vi "TimeStampToDateTimeInt.vi"(0 "Time Stamp":timestamp=timestamp(3357882633.0878906 s since 1904-01-01)) -> (1 "timeInt":u32, 2 "dateInt":u16)   [LabVIEW 2009]
panel:
  out "number":u32
  out "milliseconds":string
  out "seconds":string
  out "minute":string
  out "hour":string
  out "year":string
  out "month":string
  out "day":string
  out "time":string
  out "date":string
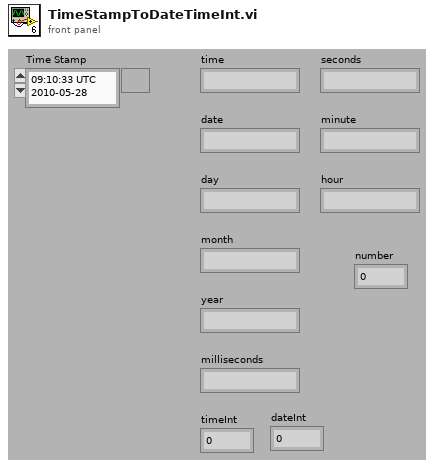
[diagram p1: front panel]
types:
  T1 = cluster{"Boolean array[0]":bool, "Boolean array[1]":bool, "Boolean array[2]":bool, "Boolean array[3]":bool, "Boolean array[4]":bool, "Boolean array[5]":bool, "Boolean array[6]":bool, "Boolean array[7]":bool, "Boolean array[8]":bool, "Boolean array[9]":bool}
  T2 = cluster{"Boolean array[0]":bool, "Boolean array[1]":bool, "Boolean array[2]":bool, "Boolean array[3]":bool, "Boolean array[4]":bool, "Boolean array[5]":bool}
  T3 = cluster{"Boolean array[0]":bool, "Boolean array[1]":bool, "Boolean array[2]":bool, "Boolean array[3]":bool, "Boolean array[4]":bool}
  T4 = cluster{"Boolean array[0]":bool, "Boolean array[1]":bool, "Boolean array[2]":bool, "Boolean array[3]":bool}
  T5 = cluster{"Boolean array[0]":bool, "Boolean array[1]":bool, "Boolean array[2]":bool, "Boolean array[3]":bool, "Boolean array[4]":bool, "Boolean array[5]":bool, "Boolean array[6]":bool}
  T6 = cluster{"Boolean array[0]":bool, "Boolean array[1]":bool, "Boolean array[2]":bool, "Boolean array[3]":bool, "Boolean array[4]":bool, "Boolean array[5]":bool, "Boolean array[6]":bool, "Boolean array[7]":bool, "Boolean array[8]":bool, "Boolean array[9]":bool, "Boolean array[0]":bool, "Boolean array[1]":bool, "Boolean array[2]":bool, "Boolean array[3]":bool, "Boolean array[4]":bool, "Boolean array[5]":bool, "Boolean array[0]":bool, "Boolean array[1]":bool, "Boolean array[2]":bool, "Boolean array[3]":bool, "Boolean array[4]":bool, "Boolean array[5]":bool, "Boolean array[0]":bool, "Boolean array[1]":bool, "Boolean array[2]":bool, "Boolean array[3]":bool, "Boolean array[4]":bool, "Boolean array[0]":bool, "Boolean array[1]":bool, "Boolean array[2]":bool, "Boolean array[3]":bool, "Boolean array[4]":bool}
  T7 = cluster{"Boolean array[0]":bool, "Boolean array[1]":bool, "Boolean array[2]":bool, "Boolean array[3]":bool, "Boolean array[4]":bool, "Boolean array[0]":bool, "Boolean array[1]":bool, "Boolean array[2]":bool, "Boolean array[3]":bool, "Boolean array[0]":bool, "Boolean array[1]":bool, "Boolean array[2]":bool, "Boolean array[3]":bool, "Boolean array[4]":bool, "Boolean array[5]":bool, "Boolean array[6]":bool}
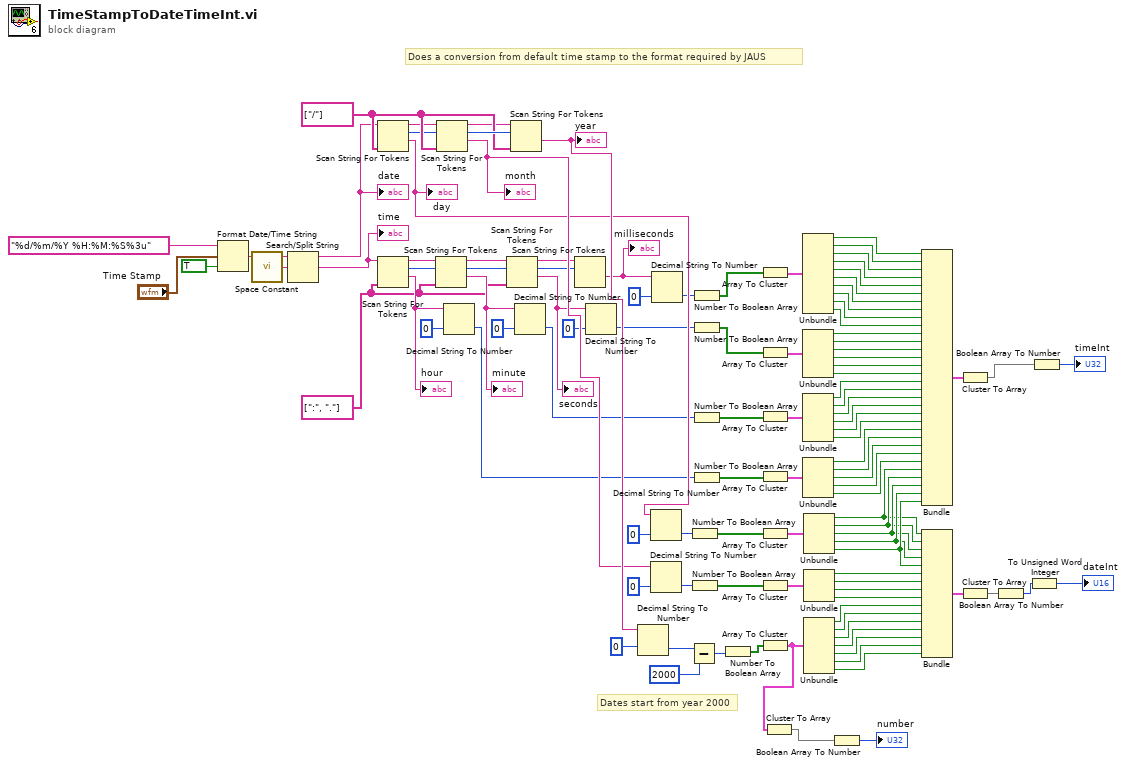
[diagram p0: block diagram]
diagram:
  w25 = string[] [":", "."] ("delimiters (\\s,\\t,\\r,\\n)")
  w18 = string[] ["/"] ("delimiters (\\s,\\t,\\r,\\n)")
  # "Dates start from year 2000"
  # "Does a conversion from default time stamp to the format required by JAUS"
  n1 = Format Date/Time String(time format string (%c)="%d/%m/%Y %H:%M:%S%3u", seconds (now)="Time Stamp", UTC format=TRUE) -> (date/time string=w12:string)
  n2 = call <vilib>:"Space Constant.vi"() -> ("String"=w13:string)
  n3 = Search/Split String(string=w12, search string/char (-)=w13) -> (substring before match=w14:string, match + rest of string=w24:string)  [unwired: 1 in, 1 out]
  "date" <- w14
  "time" <- w24
  n4 = Scan String For Tokens(6:w18, 9:w14) -> (1:w76:string, 2:w16:i32, 3:w15:string)  [unwired: 4 in, 1 out]
  "day" <- w76
  n5 = Scan String For Tokens(6:w25, 9:w24) -> (1:w28:string, 2:w21:i32, 3:w20:string)  [unwired: 4 in, 1 out]
  "hour" <- w28
  n6 = Scan String For Tokens(6:w25, 8:w21, 9:w20) -> (1:w34:string, 2:w23:i32, 3:w22:string)  [unwired: 3 in, 1 out]
  "minute" <- w34
  n7 = Scan String For Tokens(6:w18, 8:w16, 9:w15) -> (1:w91:string, 2:w19:i32, 3:w17:string)  [unwired: 3 in, 1 out]
  "month" <- w91
  n8 = Decimal String To Number(string=w28, default (0L)=u8 0 ("default (0 I32)")) -> (number=w30:u8)  [unwired: 1 in, 1 out]
  n9 = Scan String For Tokens(6:w25, 8:w23, 9:w22) -> (1:w39:string, 2:w27:i32, 3:w26:string)  [unwired: 3 in, 1 out]
  "seconds" <- w39
  n10 = Scan String For Tokens(6:w18, 8:w19, 9:w17) -> (1:w97:string)  [unwired: 3 in, 3 out]
  "year" <- w97
  n11 = Decimal String To Number(string=w34, default (0L)=u8 0 ("default (0 I32)")) -> (number=w32:u8)  [unwired: 1 in, 1 out]
  n12 = Scan String For Tokens(8:w27, 9:w26) -> (1:w43:string)  [unwired: 4 in, 3 out]
  "milliseconds" <- w43
  n13 = Decimal String To Number(string=w39, default (0L)=u8 0 ("default (0 I32)")) -> (number=w36:u8)  [unwired: 1 in, 1 out]
  n14 = Decimal String To Number(string=w97, default (0L)=u16 0 ("default (0 I32)")) -> (number=w5:u16)  [unwired: 1 in, 1 out]
  n15 = Decimal String To Number(string=w76, default (0L)=u8 0 ("default (0 I32)")) -> (number=w79:u8)  [unwired: 1 in, 1 out]
  n16 = Decimal String To Number(string=w91, default (0L)=u8 0 ("default (0 I32)")) -> (number=w90:u8)  [unwired: 1 in, 1 out]
  n17 = Decimal String To Number(string=w43, default (0L)=u16 0 ("default (0 I32)")) -> (number=w40:u16)  [unwired: 1 in, 1 out]
  n18 = Subtract(x=w5, y=u16 2000) -> (x-y=w3:u16)
  n19 = Number To Boolean Array(number=w79) -> (Boolean array=w77:bool[])
  n20 = Number To Boolean Array(number=w90) -> (Boolean array=w88:bool[])
  n21 = Number To Boolean Array(number=w40) -> (Boolean array=w41:bool[])
  n22 = Number To Boolean Array(number=w36) -> (Boolean array=w37:bool[])
  n23 = Number To Boolean Array(number=w32) -> (Boolean array=w33:bool[])
  n24 = Number To Boolean Array(number=w30) -> (Boolean array=w31:bool[])
  n25 = Number To Boolean Array(number=w3) -> (Boolean array=w2:bool[])
  n26 = Array To Cluster(array=w41) -> (cluster=w44:T1)
  n27 = Array To Cluster(array=w37) -> (cluster=w56:T2)
  n28 = Array To Cluster(array=w33) -> (cluster=w55:T2)
  n29 = Array To Cluster(array=w31) -> (cluster=w69:T3)
  n30 = Array To Cluster(array=w77) -> (cluster=w78:T3)
  n31 = Array To Cluster(array=w88) -> (cluster=w89:T4)
  n32 = Array To Cluster(array=w2) -> (cluster=w8:T5)
  n33 = Cluster To Array(cluster=w8) -> (array=w7:bool[])
  n34 = Unbundle(w44) -> ("Boolean array[0]"=w45:bool, "Boolean array[1]"=w46:bool, "Boolean array[2]"=w47:bool, "Boolean array[3]"=w48:bool, "Boolean array[4]"=w49:bool, "Boolean array[5]"=w50:bool, "Boolean array[6]"=w51:bool, "Boolean array[7]"=w52:bool, "Boolean array[8]"=w53:bool, "Boolean array[9]"=w54:bool)
  n35 = Unbundle(w56) -> ("Boolean array[0]"=w57:bool, "Boolean array[1]"=w58:bool, "Boolean array[2]"=w59:bool, "Boolean array[3]"=w60:bool, "Boolean array[4]"=w61:bool, "Boolean array[5]"=w62:bool)
  n36 = Unbundle(w55) -> ("Boolean array[0]"=w63:bool, "Boolean array[1]"=w64:bool, "Boolean array[2]"=w65:bool, "Boolean array[3]"=w66:bool, "Boolean array[4]"=w67:bool, "Boolean array[5]"=w68:bool)
  n37 = Unbundle(w69) -> ("Boolean array[0]"=w70:bool, "Boolean array[1]"=w71:bool, "Boolean array[2]"=w72:bool, "Boolean array[3]"=w73:bool, "Boolean array[4]"=w74:bool)
  n38 = Unbundle(w78) -> ("Boolean array[0]"=w82:bool, "Boolean array[1]"=w83:bool, "Boolean array[2]"=w84:bool, "Boolean array[3]"=w85:bool, "Boolean array[4]"=w86:bool)
  n39 = Unbundle(w89) -> ("Boolean array[0]"=w92:bool, "Boolean array[1]"=w93:bool, "Boolean array[2]"=w94:bool, "Boolean array[3]"=w95:bool)
  n40 = Unbundle(w8) -> ("Boolean array[0]"=w98:bool, "Boolean array[1]"=w99:bool, "Boolean array[2]"=w100:bool, "Boolean array[3]"=w101:bool, "Boolean array[4]"=w102:bool, "Boolean array[5]"=w103:bool, "Boolean array[6]"=w104:bool)
  n41 = Boolean Array To Number(Boolean array=w7) -> (number=→"number":u32)
  n42 = Bundle("Boolean array[0]"=w45, "Boolean array[1]"=w46, "Boolean array[2]"=w47, "Boolean array[3]"=w48, "Boolean array[4]"=w49, "Boolean array[5]"=w50, "Boolean array[6]"=w51, "Boolean array[7]"=w52, "Boolean array[8]"=w53, "Boolean array[9]"=w54, "Boolean array[0]"=w57, "Boolean array[1]"=w58, "Boolean array[2]"=w59, "Boolean array[3]"=w60, "Boolean array[4]"=w61, "Boolean array[5]"=w62, "Boolean array[0]"=w63, "Boolean array[1]"=w64, "Boolean array[2]"=w65, "Boolean array[3]"=w66, "Boolean array[4]"=w67, "Boolean array[5]"=w68, "Boolean array[0]"=w70, "Boolean array[1]"=w71, "Boolean array[2]"=w72, "Boolean array[3]"=w73, "Boolean array[4]"=w74, "Boolean array[0]"=w82, "Boolean array[1]"=w83, "Boolean array[2]"=w84, "Boolean array[3]"=w85, "Boolean array[4]"=w86) -> (w80:T6)  [unwired: 1 in]
  n43 = Bundle("Boolean array[0]"=w82, "Boolean array[1]"=w83, "Boolean array[2]"=w84, "Boolean array[3]"=w85, "Boolean array[4]"=w86, "Boolean array[0]"=w92, "Boolean array[1]"=w93, "Boolean array[2]"=w94, "Boolean array[3]"=w95, "Boolean array[0]"=w98, "Boolean array[1]"=w99, "Boolean array[2]"=w100, "Boolean array[3]"=w101, "Boolean array[4]"=w102, "Boolean array[5]"=w103, "Boolean array[6]"=w104) -> (w105:T7)  [unwired: 1 in]
  n44 = Cluster To Array(cluster=w80) -> (array=w81:bool[])
  n45 = Cluster To Array(cluster=w105) -> (array=w106:bool[])
  n46 = Boolean Array To Number(Boolean array=w106) -> (number=w108:u32)
  n47 = To Unsigned Word Integer(number=w108) -> (unsigned 16bit integer=→"dateInt":u16)
  n48 = Boolean Array To Number(Boolean array=w81) -> (number=→"timeInt":u32)
